vi "Do.vi"(8 "error in (no error)":errorcluster, 10 "Actor in":refnum<class "Actor.lvclass">, 11 "Conceret Initialize Msg in":refnum<class "Conceret Initialize Msg.lvclass">) -> (0 "error out":errorcluster, 2 "Actor out":refnum<class "Actor.lvclass">)   [LabVIEW 2013, in "Create Project View.lvlib" / "Conceret Initialize Msg.lvclass"]
doc: "(<B>Filename</B>: Actor Framework.lvlib:Message.lvclass:Do.vi)\n\nDefines what a message does when it is received by an actor. Generally, a message instructs an actor to invoke one of its methods.\n\nBy default, this method does nothing. A child class must override it to define behavior. Create a child class by using the Actor Framework Message Maker dialog box."
uses:
  Conceret Initialize Msg.lvclass
  <vilib>/ActorFramework/Actor/Actor.lvclass
  Create Project View/Create Project View.lvclass
  Models/Create Project Model Messages/Abstract Initialize Msg/Abstract Initialize Msg.lvclass
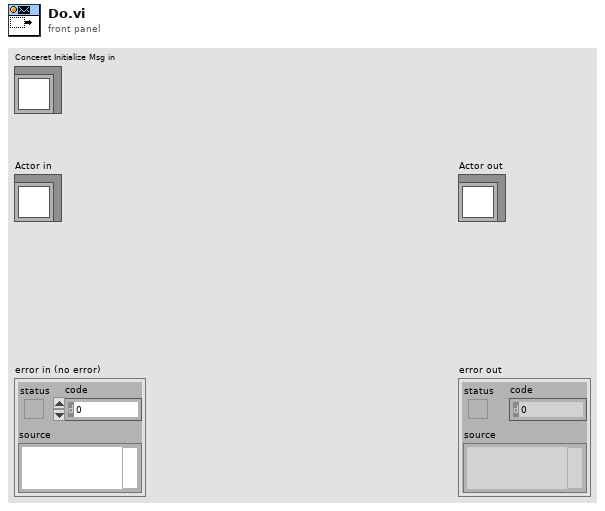
[diagram p1: front panel]
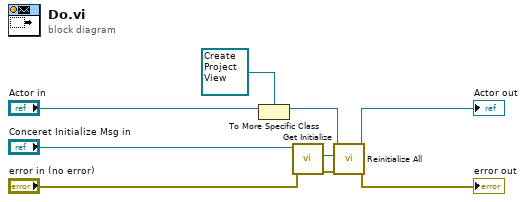
[diagram p0: block diagram]
diagram:
  n1 = To More Specific Class(target class=refnum<class "Create Project View.lvclass"> refnum ("Create Project View.lvlib:Create Project View.lvclass"), reference="Actor in") -> (specific class reference=w6:refnum<class "Create Project View.lvclass">)  [unwired: 1 in, 1 out]
  n2 = call "Get Initialize.vi"("error in (no error)"="error in (no error)", "Abstract Initialize Msg in"="Conceret Initialize Msg in") -> ("error out"=w5:errorcluster, "Initialize"=w1:bool)  [unwired: 7 in, 1 out]
  n3 = call "Reinitialize All.vi"("error in (no error)"=w5, "Initialize"=w1, "Create Project View in"=w6) -> ("error out"=→"error out":errorcluster, "Create Project View out"=→"Actor out":refnum<class "Create Project View.lvclass">)  [unwired: 7 in]
